vi "Waveform Scale and Offset.vi"(8 "error in (no error)":errorcluster, 9 "scale":dbl=1.0 format="%0.2f", 10 "offset":dbl format="%0.2f", 11 "waveform in":waveform(dbl)) -> (0 "error out":errorcluster, 3 "waveform out":waveform(dbl))   [LabVIEW 2020]
doc: "Scales the waveform data using the equation <B>waveform out</B> = (<B>scale</B> * <B>waveform in</B> + <B>offset</B>)."
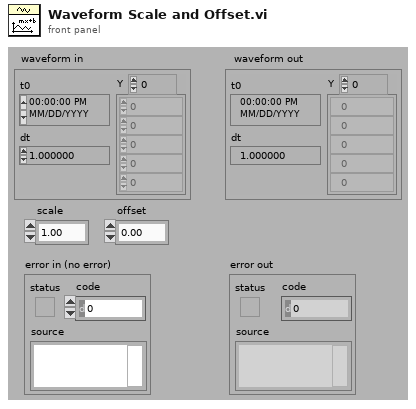
[diagram p1: front panel]
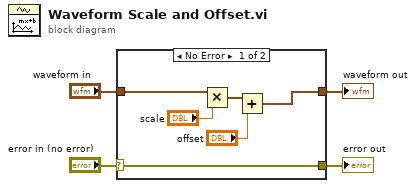
[diagram p0: block diagram]
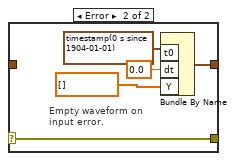
[diagram p2: hidden frame]
diagram:
  n1 = case shown="No Error" "error in (no error)" {
    selector: "error in (no error)" -> [w7 w15]
    tunnel: [w6 w14] -> w4
    tunnel: "waveform in" -> [w5 _]
    tunnel: [w7 w15] -> w1
    frame No Error {
      n2 = Multiply(x=w5, y="scale") -> (x*y=w9:waveform(dbl))
      n3 = Add(x=w9, y="offset") -> (x+y=w6:waveform(dbl))
    }
    frame Error {
      # "Empty waveform on\ninput error."
      n4 = Bundle By Name("t0"=timestamp(0 s since 1904-01-01), "dt"=0.0, "Y"=dbl[] []) -> (w14:waveform(dbl))  [unwired: 1 out]
    }
  }
  "waveform out" <- w4
  "error out" <- w1
